vi "PID Basic Tester.vi"() -> ()   [LabVIEW 2014]
panel:
  out "position":dbl
  in  "Setpoint":dbl format="%#_13g"
  out "In Range?":bool
  out "Output":dbl
  in  "stop":bool
  in  "deadband":dbl
  in  "Gains":cluster{"P":dbl, "I":dbl, "D":dbl}
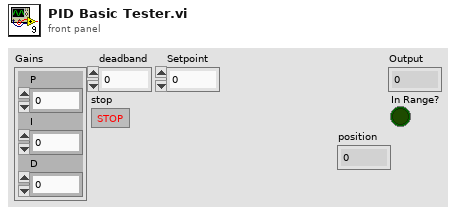
[diagram p1: front panel]
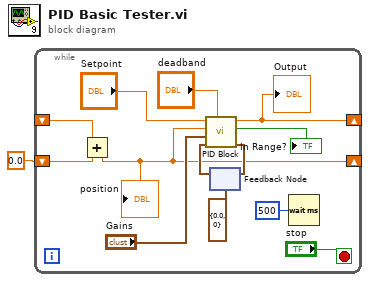
[diagram p0: block diagram]
diagram:
  n1 = while {
    shift-right: [w5] -> _
    shift-left: _ -> [w3]
    shift-right: [w4] -> _
    shift-left: 0.0 -> [w2]
    stop <- "stop" stop-if-true
    n2 = Add(x=w3, y=w2) -> (x+y=w4:dbl)
    "position" <- w4
    n3 = feedback #1(cluster{"Last Error":dbl, "Last Time":u32} {"Last Error"=0.0, "Last Time"=0} ("To Shift")) -> (w13:cluster{"Last Error":dbl, "Last Time":u32})
    n4 = call "PID Block.vi"("Deadband"="deadband", "From Shift"=w13, "Gains"="Gains", "Position"=w4, "Setpoint"="Setpoint") -> ("To Shift"=w14:cluster{"Last Error":dbl, "Last Time":u32}, "Tolerable?"=→"In Range?":bool, "Output"=w5:dbl)  [unwired: 4 in]
    "Output" <- w5
    n5 = feedback-in #1(w14) -> ()
    n6 = Wait (ms)(milliseconds to wait=u32 500) -> ()  [unwired: 1 out]
  }
